vi "Pressure_Control.vi"() -> ()   [LabVIEW 2018]
panel:
  out "Muscle Pressure 8":dynamicdata(graph)
  out "Muscle Pressure 7":dynamicdata(graph)
  out "Muscle Pressure 6":dynamicdata(graph)
  out "Muscle Pressure 5":dynamicdata(graph)
  out "Muscle Pressure 4":dynamicdata(graph)
  out "Muscle Pressure 3":dynamicdata(graph)
  out "Muscle Presure 2":dynamicdata(graph)
  in  "stop (F) 4":bool caption="stop (F)"
  out "Muscle Pressure 1":dynamicdata(graph)
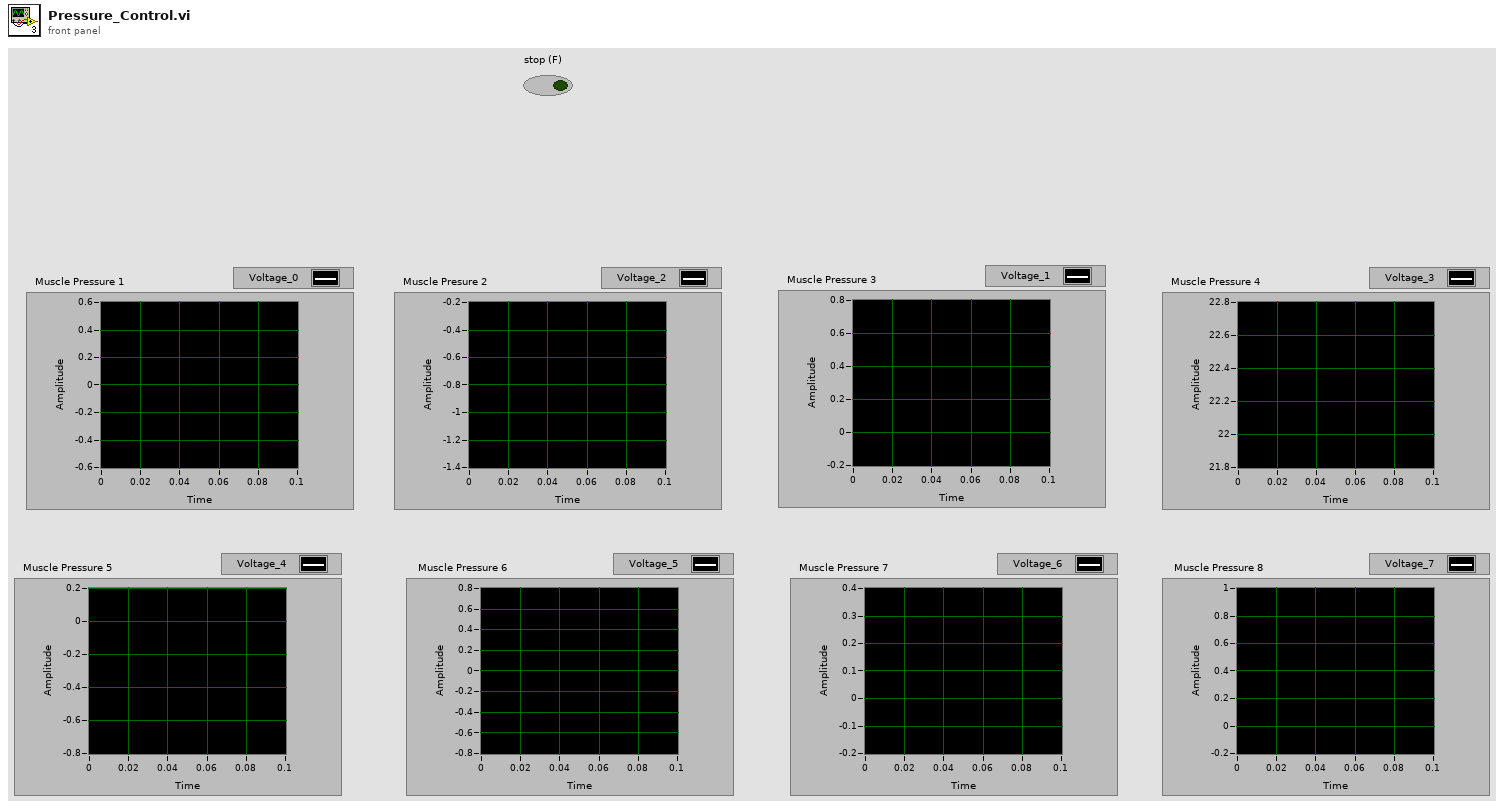
[diagram p1: front panel]
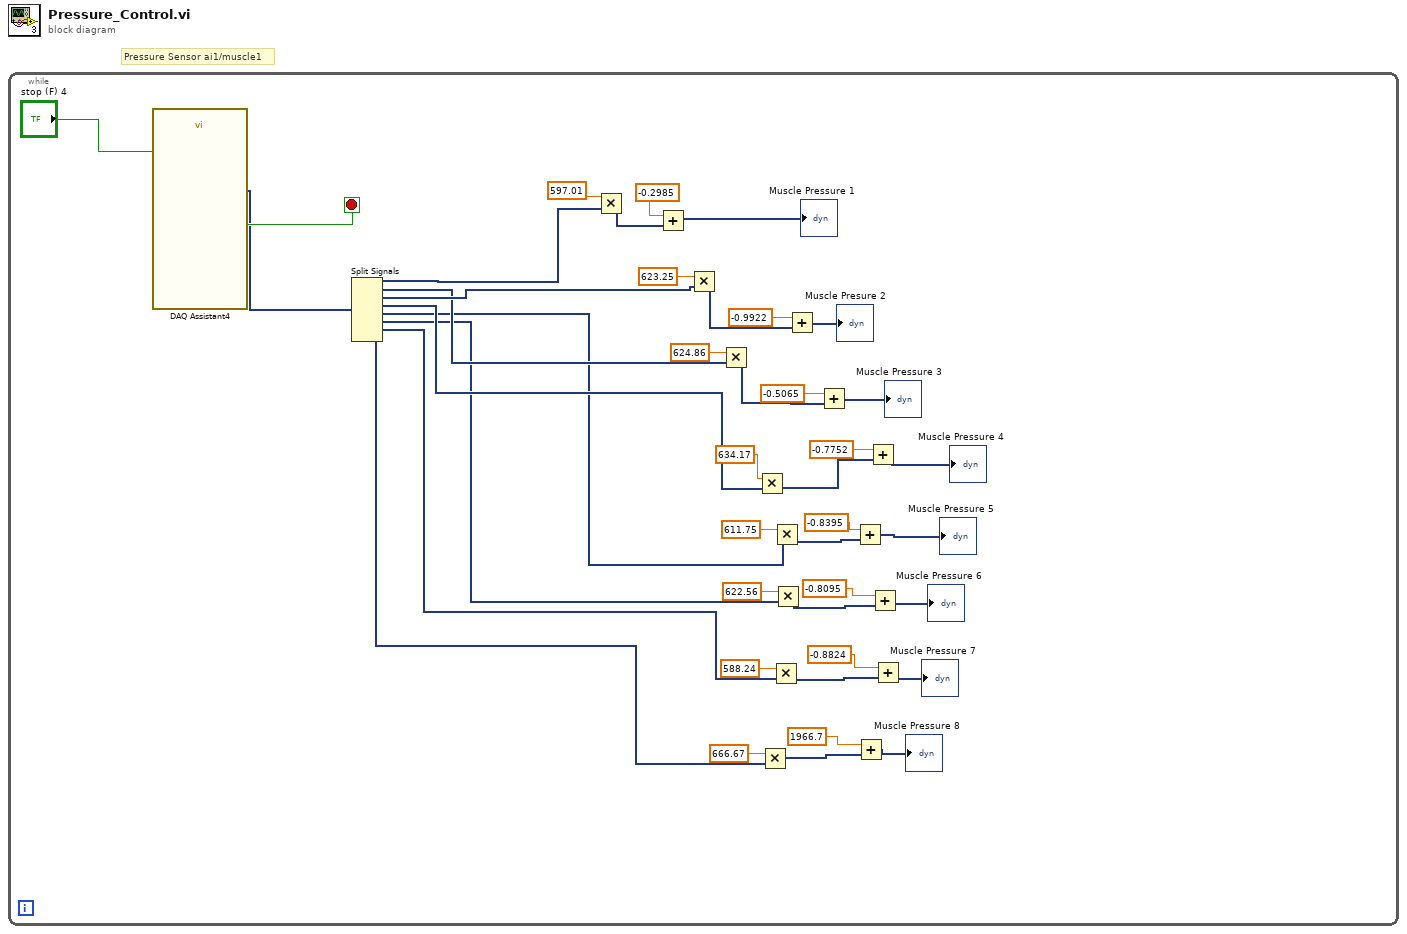
[diagram p0: block diagram]
diagram:
  # "Pressure Sensor ai1/muscle1"
  n1 = while {
    stop <- w42 stop-if-true
    n2 = call "DAQ Assistant4"("stop (F)"="stop (F) 4") -> ("data"=w26:dynamicdata, "stopped"=w42:bool)  [unwired: 15 in, 2 out]
    n3 = Split Signals(w26) -> (w28:dynamicdata, w27:dynamicdata, w29:dynamicdata, w21:dynamicdata, w16:dynamicdata, w11:dynamicdata, w6:dynamicdata, w1:dynamicdata)  [unwired: 8 in]
    n4 = Multiply(x=597.01, y=w28) -> (x*y=w38:dynamicdata)
    n5 = Add(x=-0.2985, y=w38) -> (x+y=→"Muscle Pressure 1":dynamicdata)
    n6 = Multiply(x=623.25, y=w29) -> (x*y=w37:dynamicdata)
    n7 = Multiply(x=624.86, y=w27) -> (x*y=w33:dynamicdata)
    n8 = Multiply(x=634.17, y=w21) -> (x*y=w25:dynamicdata)
    n9 = Multiply(x=666.67, y=w1) -> (x*y=w5:dynamicdata)
    n10 = Multiply(x=588.24, y=w6) -> (x*y=w10:dynamicdata)
    n11 = Multiply(x=611.75, y=w16) -> (x*y=w20:dynamicdata)
    n12 = Multiply(x=622.56, y=w11) -> (x*y=w15:dynamicdata)
    n13 = Add(x=-0.9922, y=w37) -> (x+y=→"Muscle Presure 2":dynamicdata)
    n14 = Add(x=-0.5065, y=w33) -> (x+y=→"Muscle Pressure 3":dynamicdata)
    n15 = Add(x=-0.8395, y=w20) -> (x+y=→"Muscle Pressure 5":dynamicdata)
    n16 = Add(x=1966.7, y=w5) -> (x+y=→"Muscle Pressure 8":dynamicdata)
    n17 = Add(x=-0.7752, y=w25) -> (x+y=→"Muscle Pressure 4":dynamicdata)
    n18 = Add(x=-0.8095, y=w15) -> (x+y=→"Muscle Pressure 6":dynamicdata)
    n19 = Add(x=-0.8824, y=w10) -> (x+y=→"Muscle Pressure 7":dynamicdata)
  }
